vi "SAM_Query.vi"(0 "System no.":i32=1 min=1 max=4 step=1, 2 "Axis":string[](array[string]), 5 "error in":errorcluster) -> (14 "Mode of Operations":T1[](array[typedef]), 19 "error out":errorcluster)   [LabVIEW 2020]
doc: "SAM? (Get Axis Mode)\n\nDescription\nQueries the current mode of operation of the axes.\nFor further details on the modes of operation, see \"Drive State Machine\" (p. 101). \n\nFormat\nSAM?[ <AxisID>]\n\nArguments\n<AxisID>\nAn axis of the controller\nThe available axes can be queried with USG? SYS.\nPossible values: Alias of the axis (p. 94) \n\nResponse\n{<AxisID>\"=\"<OperationMode> LF}\n3 Command Overview\nPI General Command Set (GCS) 3.0 SM160E Version: 1.0.0 55\n<OperationMode>\nMode of operation of the axis\nThe permitted modes of operation can be queried with USG? PROP (p. 79). \nThe mode of operation is specified as a decimal or hexadecimal value.\nPossible values: See list of modes of operation (p. 102) \n\nExample\nSee SAM (p. 52) for an example.\n\nNotes\nThe current mode of operation is also displayed in the status register of the axis (p. 97). The \nstatus register can be queried with the STV? command (p. 66). \nThe current mode of operation of an axis can be set with the SAM command. \n\nUser command level\nUSR"
uses:
  ModeOfOperation.ctl
panel:
  # "SAM? (Get Axis Mode)\n\nQueries the current mode of operation of the axes.\nFor further details on the modes of operation, see \"Drive State Machine\"."
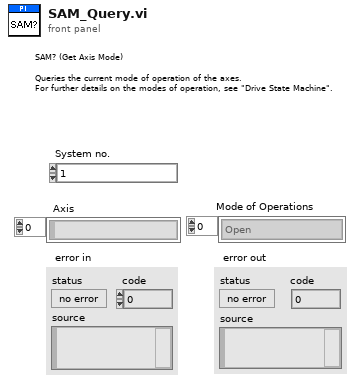
[diagram p1: front panel]
types:
  T1 = typedef "ModeOfOperation.ctl" = enum16{"Open", "Open-Loop Position", "Closed-Loop Position", "Open-Loop Velocity", "Closed-Loop Velocity", "Open-Loop Force", "Closed-Loop Force", "Step Operation"}
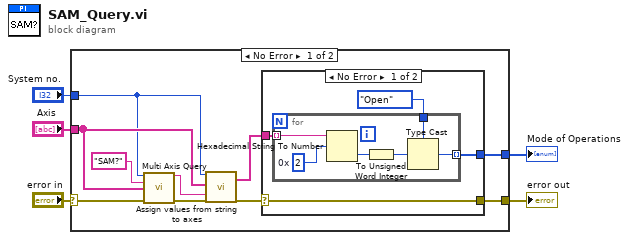
[diagram p0: block diagram]
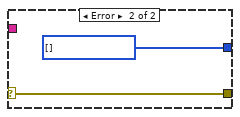
[diagram p2: hidden frame]
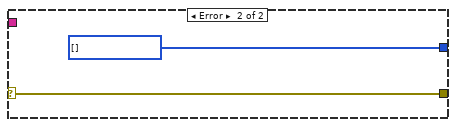
[diagram p3: hidden frame]
diagram:
  n1 = case shown="No Error" "error in" {
    selector: "error in" -> [w14 w29]
    tunnel: [w7 w29] -> w5
    tunnel: "Axis" -> [w11 _]
    tunnel: "System no." -> [w10 _]
    tunnel: [w8 w28] -> w1
    frame No Error {
      n2 = call "Multi Axis Query.vi"("System no."=w10, "Command"="SAM?", "Axis"=w11, "error in (no error)"=w14) -> ("Answer"=w13:string, "error out"=w12:errorcluster)  [unwired: 10 in]
      n3 = call "Assign values from string to axes.vi"("System no."=w10, "Queried axes"=w11, "Input String"=w13, "error in"=w12) -> ("Strings"=w9:string[], "error out"=w6:errorcluster)  [unwired: 2 in, 12 out]
      n4 = case shown="No Error" w6 {
        selector: w6 -> [w17 w27]
        tunnel: w9 -> [w19 _]
        tunnel: [w18 w26] -> w8
        tunnel: [w17 w27] -> w7
        frame No Error {
          n5 = for {
            tunnel: w19 -> [w23] mode=indexing
            tunnel: ModeOfOperation."Open" ("Drive State") -> [w25]
            tunnel: [w24] -> w18 mode=indexing
            w22 = 2  # 0x
            n6 = Hexadecimal String To Number(string=w23, offset=w22) -> (number=w21:u32)  [unwired: 1 in, 1 out]
            n7 = To Unsigned Word Integer(number=w21) -> (unsigned 16bit integer=w20:u16)
            n8 = Type Cast(type=w25, x=w20) -> (*(type *) &x=w24:T1)
          }
        }
        frame Error {
          w26 = T1[] [] items=["Open", "Open-Loop Position", "Closed-Loop Position", "Open-Loop Velocity", "Closed-Loop Velocity", "Open-Loop Force", "Closed-Loop Force", "Step Operation"]
        }
      }
    }
    frame Error {
      w28 = T1[] [] items=["Open", "Open-Loop Position", "Closed-Loop Position", "Open-Loop Velocity", "Closed-Loop Velocity", "Open-Loop Force", "Closed-Loop Force", "Step Operation"]
    }
  }
  "error out" <- w5
  "Mode of Operations" <- w1
